vi "Get Number HS Speeds.vi"(8 "error in (no error)":errorcluster, 9 "speeds":i32, 10 "typ":i32, 11 "channel":i32) -> (0 "error out":errorcluster, 1 "speeds out":i32, 3 "function return":u32)   [LabVIEW 2014, in "atmcd32d.lvlib"]
doc: "unsigned int WINAPI GetNumberHSSpeeds(int channel, int typ, int * speeds);"
uses:
  atmcd32d.lvlib
  atmcd32d.dll
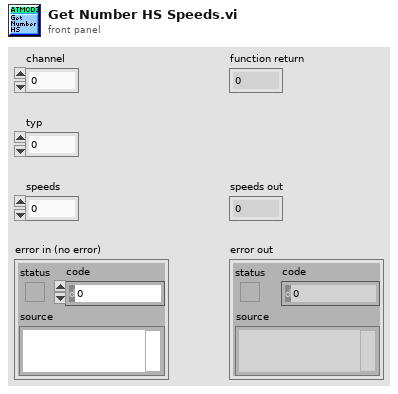
[diagram p1: front panel]
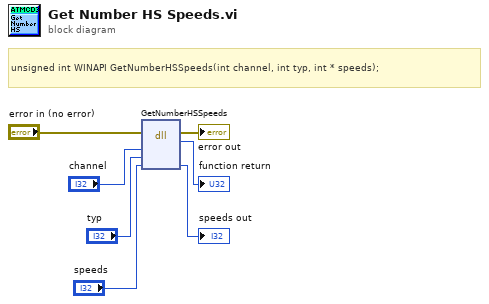
[diagram p0: block diagram]
diagram:
  # "unsigned int WINAPI GetNumberHSSpeeds(int channel, int typ, int * speeds);"
  n1 = dll-call lib="C:/Users/Bakir/Documents/Lambda2-Testing/lib/Andorlib/atmcd32d.*" fn="GetNumberHSSpeeds"(error in="error in (no error)", "channel"="channel", "typ"="typ", "speeds"="speeds") -> (error out=→"error out":errorcluster, →"function return":u32, "speeds"=→"speeds out":i32)  [unwired: 4 in, 1 out]
